vi "ma_SML Peak-hold Averaging (complex input).vi"(0 "x":cdb[](array[numeric]) format="%.2f", 1 "reset?":bool) -> (2 "y":cdb[](array[numeric]) format="%.2f", 3 "averages sofar":dbl, 4 "data ready?":bool)   [LabVIEW 2020, in "NI_MAPro.lvlib"]
uses:
  NI_MAPro.lvlib
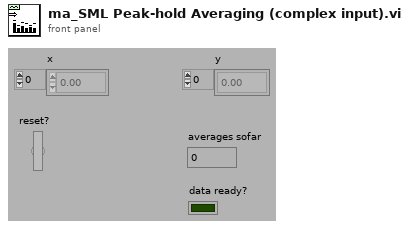
[diagram p1: front panel]
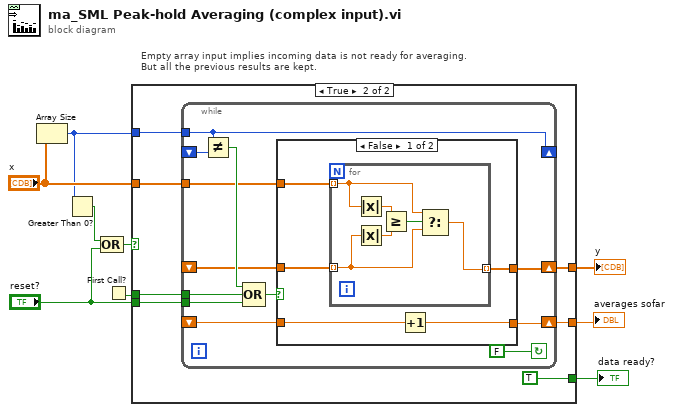
[diagram p0: block diagram]
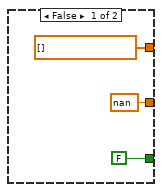
[diagram p2: hidden frame]
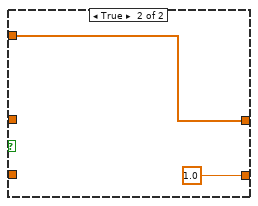
[diagram p3: hidden frame]
diagram:
  # "Empty array input implies incoming data is not ready for averaging.\nBut all the previous results are kept."
  n1 = Array Size(array="x") -> (size(s)=w4:i32)
  n2 = Greater Than 0?(x=w4) -> (x > 0?=w6:bool)
  n3 = Compound Arithmetic op=OR(w6, "reset?") -> (w5:bool)
  n4 = First Call?() -> (First Call?: T/F=w1:bool)
  n5 = case shown="True" w5 {
    tunnel: "x" -> [_ w19]
    tunnel: w4 -> [_ w18]
    tunnel: "reset?" -> [_ w17]
    tunnel: [cdb[] [] ("x") w16] -> w8
    tunnel: [nan w15] -> w7
    tunnel: [FALSE TRUE] -> w3
    tunnel: w1 -> [_ w13]
    frame False {
    }
    frame True {
      n6 = while {
        tunnel: w13 -> [w20]
        shift-left: _ -> [w22]
        shift-right: [w23] -> w15
        shift-left: _ -> [w24]
        shift-right: [w25] -> w16
        tunnel: w17 -> [w28]
        tunnel: w18 -> [w27]
        tunnel: w19 -> [w26]
        shift-left: _ -> [w30]
        shift-right: [w27] -> _
        stop <- FALSE continue-if-true
        n7 = Not Equal?(x=w27, y=w30) -> (x != y?=w29:bool)
        n8 = Compound Arithmetic op=OR(w29, w20, w28) -> (w31:bool)
        n9 = case shown="False" w31 {
          tunnel: [w34 w44] -> w25
          tunnel: w26 -> [w36 w44]
          tunnel: w24 -> [w35 _]
          tunnel: [w32 1.0] -> w23
          tunnel: w22 -> [w33 _]
          frame False {
            n10 = for {
              tunnel: w36 -> [w39] mode=indexing
              tunnel: w35 -> [w38] mode=indexing
              tunnel: [w37] -> w34 mode=indexing
              n11 = Absolute Value(x=w39) -> (abs(x)=w42:dbl)
              n12 = Absolute Value(x=w38) -> (abs(x)=w41:dbl)
              n13 = Greater Or Equal?(x=w42, y=w41) -> (x >= y?=w40:bool)
              n14 = Select(t=w39, s=w40, f=w38) -> (s? t:f=w37:cdb)
            }
            n15 = Increment(x=w33) -> (x+1=w32:dbl)
          }
          frame True {
          }
        }
      }
    }
  }
  "y" <- w8
  "averages sofar" <- w7
  "data ready?" <- w3
